vi "soc_check.vi"(1 "SoC":u16) -> (0 "SoC":dbl)   [LabVIEW 2021]
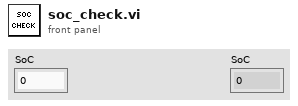
[diagram p1: front panel]
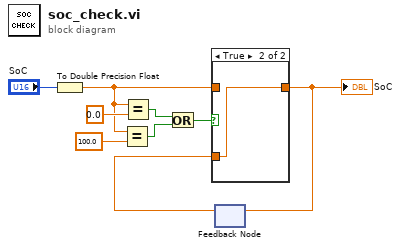
[diagram p0: block diagram]
diagram:
  n1 = To Double Precision Float(number="SoC") -> (double precision float=w4:dbl)
  n2 = Equal?(x=w4, y=100.0) -> (x = y?=w2:bool)
  n3 = Equal?(x=w4, y=0.0) -> (x = y?=w3:bool)
  n4 = Or(x=w3, y=w2) -> (x .or. y?=w1:bool)
  n5 = feedback #1() -> (w7:dbl)  [unwired: 1 in]
  n6 = case shown="True" w1 {
    tunnel: w4 -> [w10 _]
    tunnel: [w10 w11] -> w9
    tunnel: w7 -> [_ w11]
    frame False {
    }
    frame True {
    }
  }
  "SoC" <- w9
  n7 = feedback-in #1(w9) -> ()
